vi "Static Ctor.vi"(8 "error in (no error)":errorcluster, 10 "Display-As":string, 11 "Panel in":refnum<class "Panel.lvclass">) -> (0 "error out":errorcluster, 3 "Panel out":refnum<class "Panel.lvclass">)   [LabVIEW 2020, in "OOPanel.lvlib" / "Panel.lvclass"]
uses:
  Panel.lvclass
  Visbility Event Data.ctl
  Visibility State.ctl
  Close Reason.ctl
  Panel.lvclass/Panel.ctl
  OOPanel.lvlib
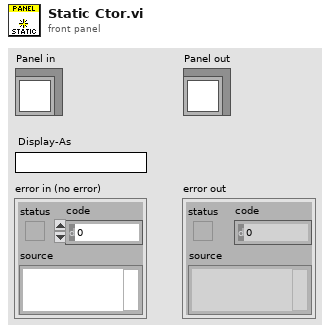
[diagram p1: front panel]
types:
  T1 = typedef "OOPanel.lvlib/Close Reason.ctl" = enum16{"Shutdown", "Close"}
  T2 = typedef "OOPanel.lvlib/Panel.lvclass/Visbility Event Data.ctl" = cluster{"State":T3}
  T3 = typedef "OOPanel.lvlib/Visibility State.ctl" = enum16{"Idle", "Closed", "Hidden", "Visible", "Subpanel"}
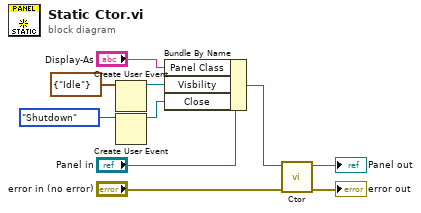
[diagram p0: block diagram]
diagram:
  n1 = Create User Event(user event datatype=T2 {"State"=enum."Idle"} ("Visible")) -> (user event=w3:refnum<user-event>)  [unwired: 1 in, 1 out]
  n2 = Create User Event(user event datatype=Close_Reason."Shutdown" ("Reason")) -> (user event=w2:refnum<user-event>)  [unwired: 1 in, 1 out]
  n3 = Bundle By Name(cluster="Panel in", "Panel Class"="Display-As", "Visbility"=w3, "Close"=w2) -> (w4:refnum<class "Panel.lvclass">)
  n4 = call-dynamic "Ctor.vi"("error in (no error)"="error in (no error)", "Panel in"=w4) -> ("error out"=→"error out":errorcluster, "Panel out"=→"Panel out":refnum<class "Panel.lvclass">)  [unwired: 8 in]
